vi "Helmholtz2D_FEM_Init Data_Coef Mtrx.vi"(11 "# of unknown":i32) -> (3 "Coef Mtrx":T1)   [LabVIEW 2020, in "NI_PDE.lvlib"]
uses:
  <vilib>/gmath/NI_PDE.lvlib
  <vilib>/gmath/pde.llb/Common/PDE_Sparse Mtrx.ctl
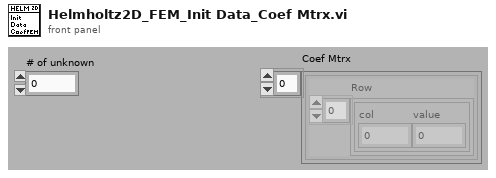
[diagram p1: front panel]
types:
  T1 = typedef "NI_PDE.lvlib/PDE_Sparse Mtrx.ctl" = cluster{"Row":cluster{"col":i32, "value":dbl}[]}[]
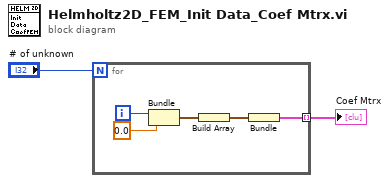
[diagram p0: block diagram]
diagram:
  n1 = for {
    N: "# of unknown" -> [_]
    tunnel: [w3] -> w1 mode=indexing
    i -> [w7]
    n2 = Bundle(w7, "value"=0.0) -> (w5:cluster{i32, "value":dbl})  [unwired: 1 out]
    n3 = Build Array(w5) -> (w4:cluster{i32, "value":dbl}[])
    n4 = Bundle(w4) -> (w3:cluster{cluster{i32, "value":dbl}[]})  [unwired: 1 in]
  }
  "Coef Mtrx" <- w1
